vi "DeInit.vi"(8 "error in (no error)":errorcluster, 11 "Jiaxin_Stepper_Controller in":refnum<class "Jiaxin_Stepper_Controller.lvclass">) -> (0 "error out":errorcluster, 3 "Jiaxin_Stepper_Controller out":refnum<class "Jiaxin_Stepper_Controller.lvclass">)   [LabVIEW 2023, in "Jiaxin_Stepper_Controller.lvlib" / "Jiaxin_Stepper_Controller.lvclass"]
uses:
  Jiaxin_Stepper_Controller.lvclass
  Jiaxin_Stepper_Controller.lvclass/Jiaxin_Stepper_Controller.ctl
  Plasmionique/MB Master/MB_Master/MB_Master.lvclass
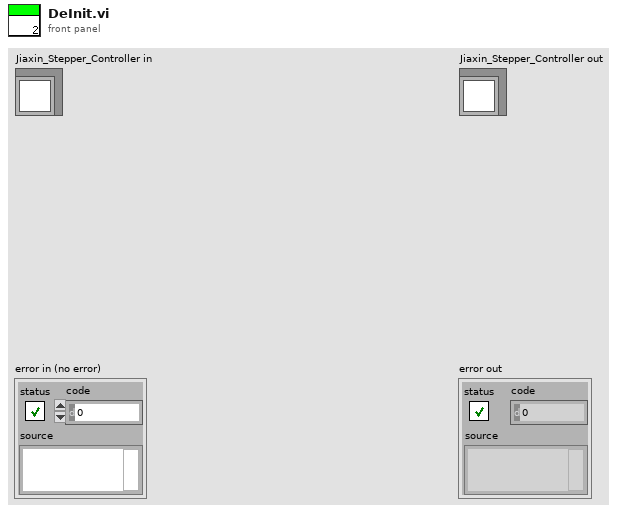
[diagram p1: front panel]
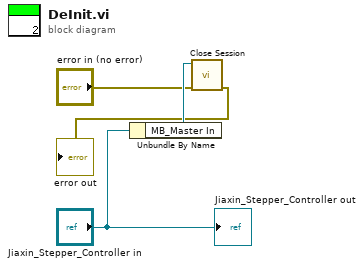
[diagram p0: block diagram]
diagram:
  n1 = Unbundle By Name("Jiaxin_Stepper_Controller in") -> ("MB_Master In"=w4:refnum<class "MB_Master.lvclass">)
  n2 = call-dynamic "Close Session.vi"("error in (no error)"="error in (no error)", "MB session in"=w4) -> ("error out"=→"error out":errorcluster)  [unwired: 9 in]
  "Jiaxin_Stepper_Controller out" <- "Jiaxin_Stepper_Controller in"
